vi "WillDey_Channels.vi"() -> ()   [LabVIEW 2017]
panel:
  in  "DC Power Supply":refnum<k15>
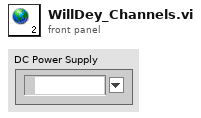
[diagram p1: front panel]
diagram:
